vi "Cam # AE.vi"(7 "Update?":bool, 11 "Ball # In":i32) -> (3 "Ball # Out":i32)   [LabVIEW 2023]
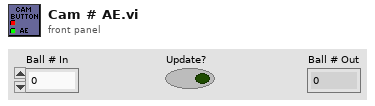
[diagram p1: front panel]
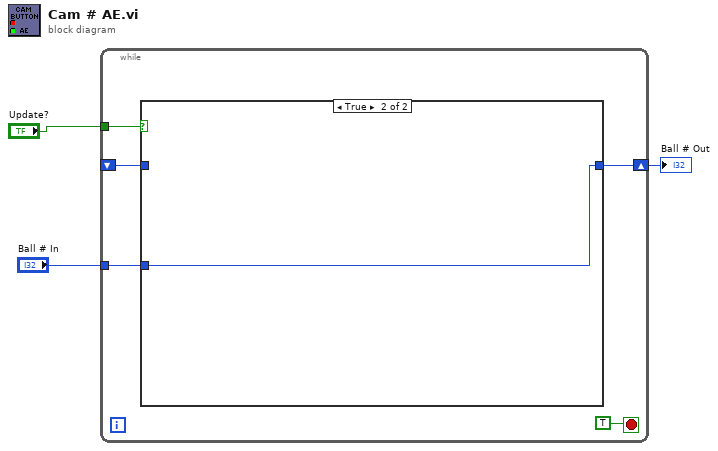
[diagram p0: block diagram]
diagram:
  n1 = while {
    shift-right: [w5] -> w1
    shift-left: _ -> [w6]
    tunnel: "Update?" -> [w7]
    tunnel: "Ball # In" -> [w4]
    stop <- TRUE stop-if-true
    n2 = case shown="True" w7 {
      tunnel: [w9 w10] -> w5
      tunnel: w6 -> [w9 _]
      tunnel: w4 -> [_ w10]
      frame False {
      }
      frame True {
      }
    }
  }
  "Ball # Out" <- w1
